vi "未命名 3.vi"() -> ()   [LabVIEW 2016]
panel:
  out "长度":i32
  out "trimmed string":string caption="删减后字符串"
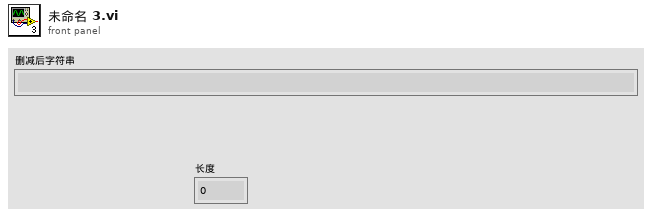
[diagram p1: front panel]
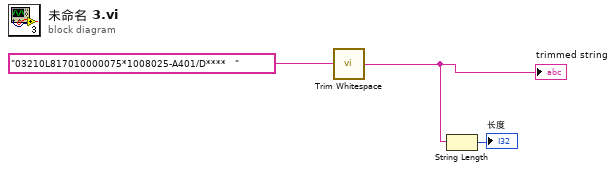
[diagram p0: block diagram]
diagram:
  n1 = call <vilib>:"Trim Whitespace.vi"("string"="03210L817010000075*1008025-A401/D****   " ("Barcode")) -> ("trimmed string"=w2:string)  [unwired: 1 in]
  "trimmed string" <- w2
  n2 = String Length(string=w2) -> (length=→"长度":i32)
